vi "Query Slot.vi"(8 "error in (no error)":errorcluster, 9 "Slot Number(0: slot 1)":i32(ring) items=["slot 1", "slot 2"], 11 "VISA resource name":refnum<visa-resource-name>) -> (0 "error out":errorcluster, 2 "Real Card In Slot":bool, 3 "VISA resource name out":refnum<visa-resource-name>)   [LabVIEW 2023, in "Keithley DMM6500 DAQ6500 Series.lvlib"]
doc: "Queries if there's any real card in specific slot."
uses:
  <instrlib>/Keithley DMM6500 DAQ6500 Series/Keithley DMM6500 DAQ6500 Series.lvlib
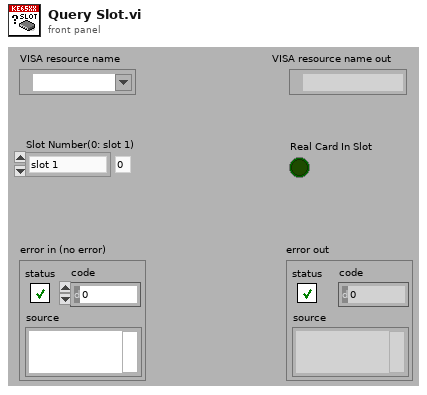
[diagram p1: front panel]
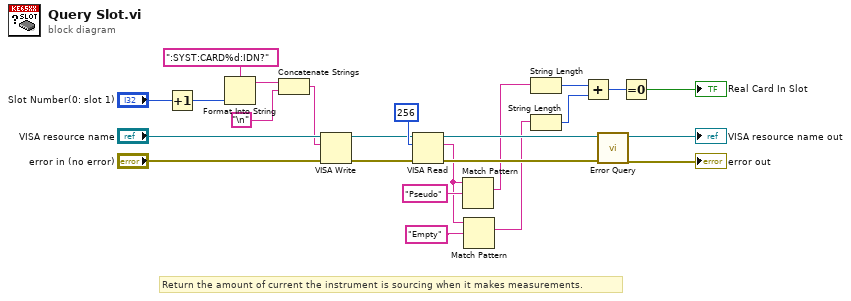
[diagram p0: block diagram]
diagram:
  # "Return the amount of current the instrument is sourcing when it makes measurements."
  n1 = Increment(x="Slot Number(0: slot 1)") -> (x+1=w7:i32)
  n2 = Format Into String(format string=":SYST:CARD%d:IDN?", w7) -> (resulting string=w9:string)  [unwired: 2 in, 1 out]
  n3 = Concatenate Strings(w9, "\n") -> (w13:string)
  n4 = VISA Write(VISA resource name="VISA resource name", write buffer=w13, error in (no error)="error in (no error)") -> (VISA resource name out=w18:refnum<visa-resource-name>, error out=w21:errorcluster)  [unwired: 1 out]
  n5 = VISA Read(VISA resource name=w18, byte count=u32 256, error in (no error)=w21) -> (VISA resource name out=w17:refnum<visa-resource-name>, read buffer=w6:string, error out=w20:errorcluster)  [unwired: 1 out]
  n6 = Match Pattern(string=w6, regular expression="Pseudo") -> (match substring=w12:string)  [unwired: 1 in, 3 out]
  n7 = Match Pattern(string=w6, regular expression="Empty") -> (match substring=w3:string)  [unwired: 1 in, 3 out]
  n8 = String Length(string=w12) -> (length=w1:i32)
  n9 = String Length(string=w3) -> (length=w2:i32)
  n10 = Add(x=w1, y=w2) -> (x+y=w4:i32)
  n11 = call <instrlib>:"Error Query.vi"("error in (no error)"=w20, "VISA resource name"=w17) -> ("error out"=→"error out":errorcluster, "VISA resource name out"=→"VISA resource name out":refnum<visa-resource-name>)  [unwired: 6 in, 2 out]
  n12 = Equal To 0?(x=w4) -> (x = 0?=→"Real Card In Slot":bool)
